vi "ConfigParams - Set - UDPConfig.vi"(8 "error in (no error)":errorcluster, 9 "UDPConfigPeriod_mS":i32=1000, 10 "UDP Config Port":i32=58431, 11 "Ethernet in":refnum<class "ENET_BS1201.lvclass">) -> (0 "error out":errorcluster, 3 "Ethernet out":refnum<class "ENET_BS1201.lvclass">)   [LabVIEW 2021, in "BS120x Driver.lvlib" / "ENET_BS1201.lvclass"]
uses:
  ENET_BS1201.lvclass
panel:
  # "[UDPConfig]\nUDPConfigPort = 58431\nUDPConfigPeriod_mS = 1000"
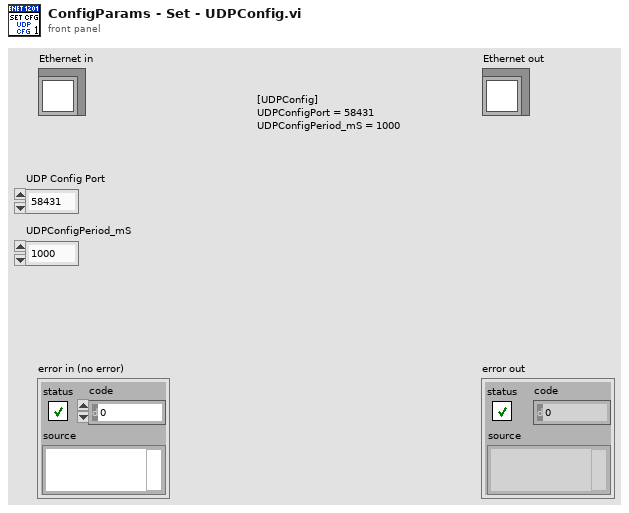
[diagram p1: front panel]
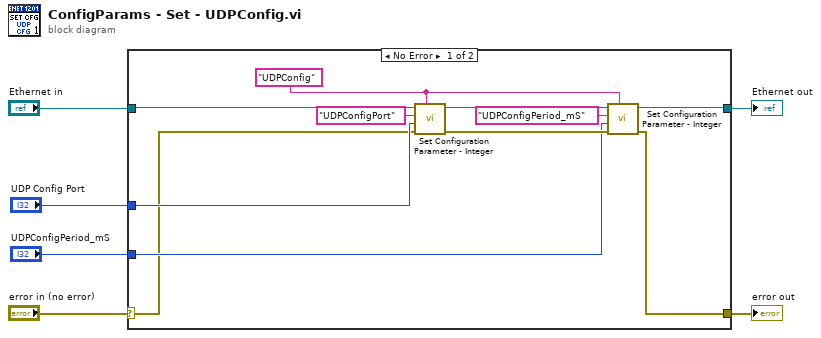
[diagram p0: block diagram]
diagram:
  n1 = case shown="No Error" "error in (no error)" {
    selector: "error in (no error)" -> [w7 w19]
    tunnel: [w9 w19] -> w5
    tunnel: [w10 w18] -> w3
    tunnel: "Ethernet in" -> [w8 w18]
    tunnel: "UDP Config Port" -> [w16 _]
    tunnel: "UDPConfigPeriod_mS" -> [w11 _]
    frame No Error {
      w13 = "UDPConfig" ("Section")
      n2 = call-dynamic "Set Configuration Parameter - Integer.vi"("Section"=w13, "error in (no error)"=w7, "Value"=w16, "Key"="UDPConfigPort", "Ethernet in"=w8) -> ("error out"=w14:errorcluster, "Ethernet out"=w15:refnum<class "ENET_BS1201.lvclass">)  [unwired: 5 in]
      n3 = call-dynamic "Set Configuration Parameter - Integer.vi"("Section"=w13, "error in (no error)"=w14, "Value"=w11, "Key"="UDPConfigPeriod_mS", "Ethernet in"=w15) -> ("error out"=w9:errorcluster, "Ethernet out"=w10:refnum<class "ENET_BS1201.lvclass">)  [unwired: 5 in]
    }
    frame Error {
    }
  }
  "error out" <- w5
  "Ethernet out" <- w3
